vi "setUp.vi"(8 "error in (no error)":errorcluster, 11 "reference in":refnum<class "Test-File IO.lvclass">) -> (0 "error out":errorcluster, 3 "reference out":refnum<class "Test-File IO.lvclass">)   [LabVIEW 2019, in "Test-File IO.lvclass"]
doc: "setUp runs prior to the test method during test execution. Use this method to initialize any object data required by your tests."
uses:
  Test-File IO.lvclass
  C:/Program Files (x86)/National Instruments/LabVIEW 2019/vi.lib/addons/_JKI Toolkits/VI Tester/TestCase.llb/TestCase.lvclass
  Test-File IO.lvclass/Test-File IO.ctl
  <vilib>/addons/_JKI Toolkits/VI Tester/TestCase.llb/TestCase.lvclass
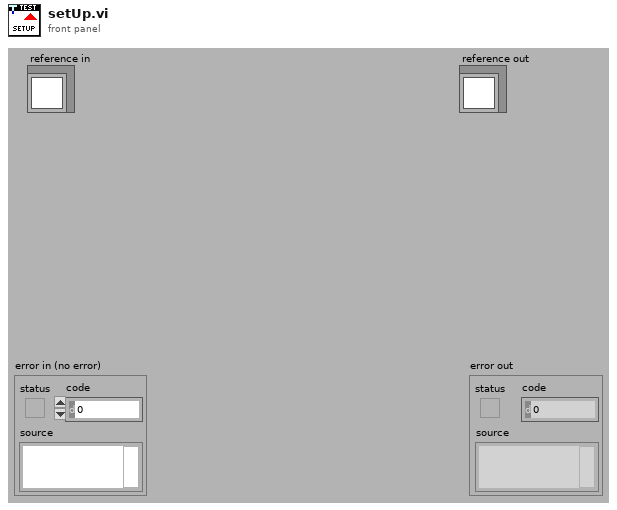
[diagram p1: front panel]
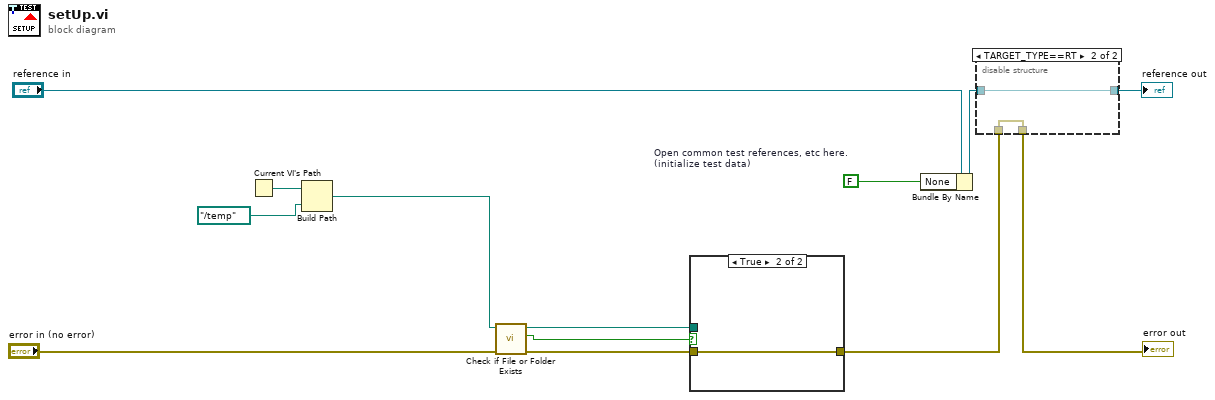
[diagram p0: block diagram]
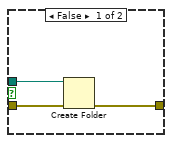
[diagram p2: hidden frame]
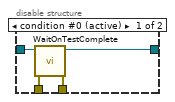
[diagram p3: hidden frame]
diagram:
  w8 = FALSE  # Open common test references, etc here. (initialize test data)
  n1 = Current VI's Path() -> (path=w7:path)
  n2 = Build Path(base path=w7, name or relative path=path "../temp") -> (appended path=w4:path)
  n3 = call <vilib>:"Check if File or Folder Exists.vi"("error in (no error)"="error in (no error)", "path"=w4) -> ("error out"=w5:errorcluster, "file or folder exists?"=w1:bool, "dup path"=w2:path)  [unwired: 7 in]
  n4 = case shown="True" w1 {
    tunnel: w5 -> [w16 w17]
    tunnel: [w15 w17] -> w3
    tunnel: w2 -> [w14 _]
    frame False {
      n5 = Create Folder(path (use dialog)=w14, error in=w16) -> (error out=w15:errorcluster)  [unwired: 1 in, 2 out]
    }
    frame True {
    }
  }
  n6 = Bundle By Name(cluster="reference in", "None"=w8) -> (w9:refnum<class "Test-File IO.lvclass">)
  n7 = disable-structure shown="TARGET_TYPE==RT" {
    disable-tunnel: w3 -> [w21 w22]
    disable-tunnel: [w20 w22] -> w12
    disable-tunnel: [w19 w23] -> w10
    disable-tunnel: w9 -> [w18 w23]
    frame condition #0 (active) {
      n8 = call <vilib>:"WaitOnTestComplete.vi"("error in (no error)"=w21, "TestCase in"=w18) -> ("error out"=w20:errorcluster, "TestCase out"=w19:refnum<class "Test-File IO.lvclass">)  [unwired: 8 in]
    }
    frame condition #1 {
    }
  }
  "error out" <- w12
  "reference out" <- w10
